vi "Client Single Connection.vi"() -> ()   [LabVIEW 2020]
doc: "This WebSockets API example VI acts as a client to make an outgoing websockets connection. Receives/sends string data to the connected server.\nWebSockets 2.0.1.40\nSam Sharp - MediaMongrels Ltd\nCopyright (c) 2019, MediaMongrels Ltd"
uses:
  <vilib>/MediaMongrels Ltd/WebSockets/WebSockets/WebSocket/WebSocket.lvclass/WebSocket.ctl
  <vilib>/MediaMongrels Ltd/WebSockets/WebSockets/WebSocket Client/WebSocket Client.lvclass
  C:/Program Files (x86)/National Instruments/LabVIEW 2020/vi.lib/MediaMongrels Ltd/WebSockets/WebSockets/WebSocket/WebSocket.lvclass
  <vilib>/MediaMongrels Ltd/WebSockets/WebSockets/WebSocket/WebSocket.lvclass
  <vilib>/addons/_JKI.lib/Serialization/JSON/JKI JSON Serialization.lvlib
panel:
  out "value":string
  in  "path":string[](array[string])
  in  "data":variant caption="Data"
  in  "command":string caption="Command"
  in  "Disconnect":bool
  in  "Connect":bool
  in  "WebSockets URL":string="ws://IP Address:Port"
  out "HTTP Headers":variant
  in  "Stop":bool
  out "Received Data":string
  in  "Send":bool
  # "WebSockets Client Example"
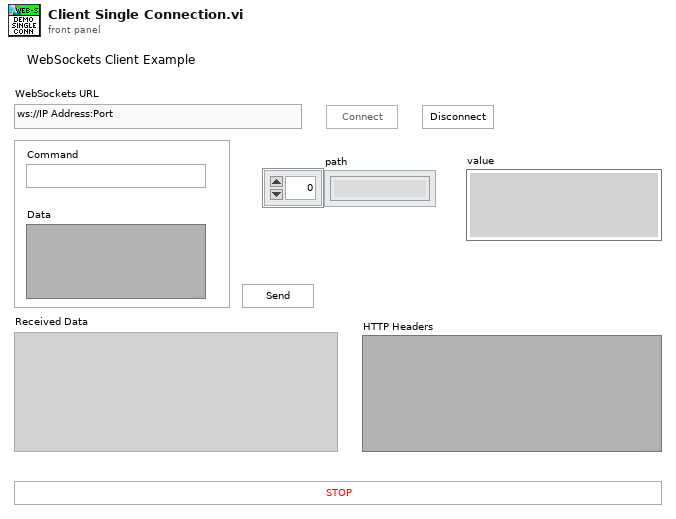
[diagram p1: front panel]
types:
  T1 = enum8{"Enabled", "Disabled", "Disabled and Grayed Out"}
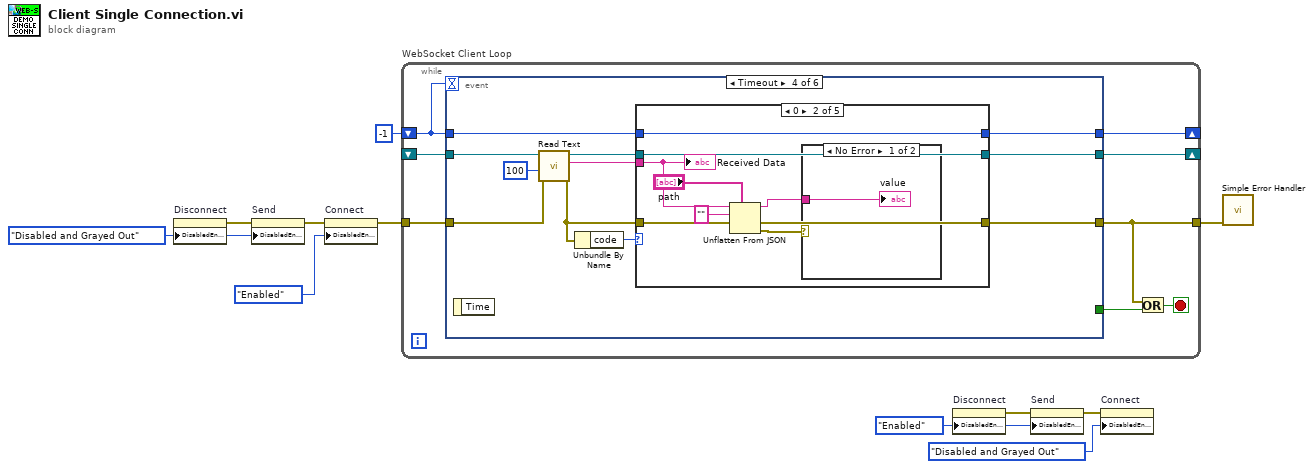
[diagram p0: block diagram]
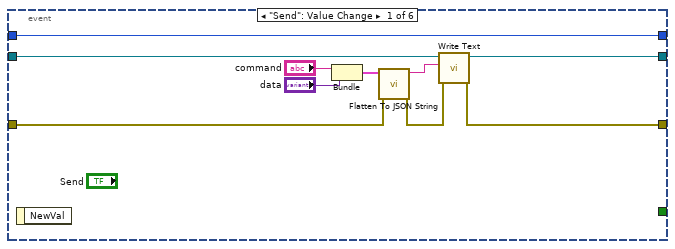
[diagram p2: hidden frame]
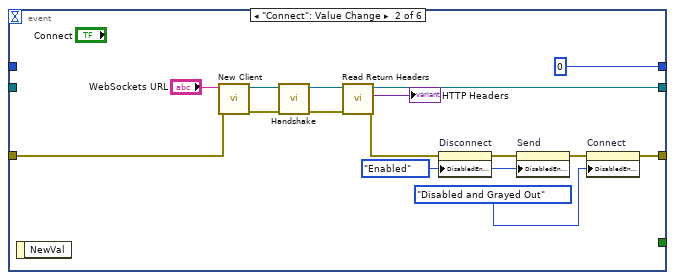
[diagram p3: hidden frame]
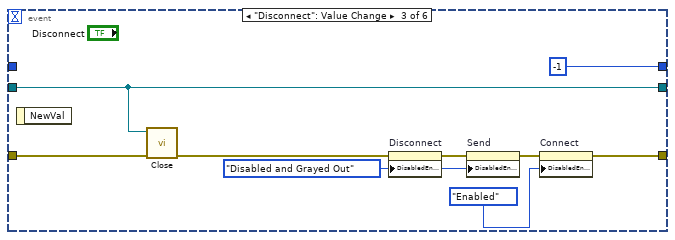
[diagram p4: hidden frame]
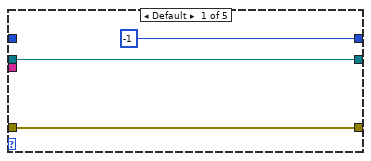
[diagram p5: hidden frame]
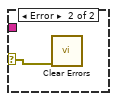
[diagram p6: hidden frame]
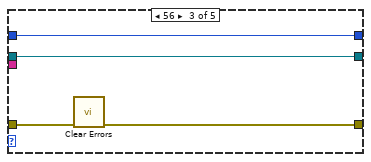
[diagram p7: hidden frame]
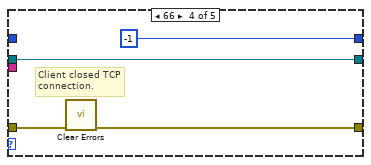
[diagram p8: hidden frame]
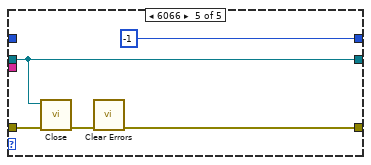
[diagram p9: hidden frame]
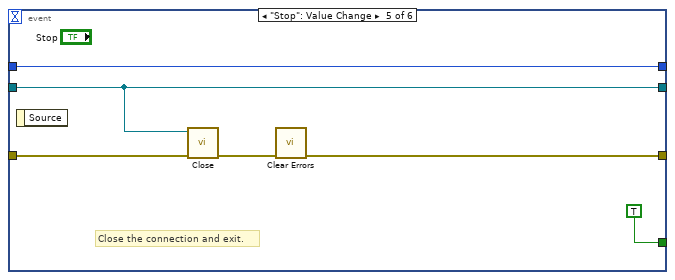
[diagram p10: hidden frame]
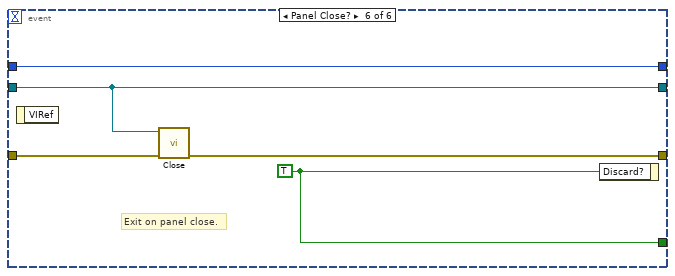
[diagram p11: hidden frame]
diagram:
  w4 = T1."Enabled" ("Disabled")
  w8 = T1."Disabled and Grayed Out" ("Disabled")
  n1 = property on="Disconnect" class="Bool"("DisabledEnum"=w8) -> (error out=w9:errorcluster)  [unwired: 2 in, 1 out]
  n2 = property on="Send" class="Bool"(error in=w9, "DisabledEnum"=w8) -> (error out=w3:errorcluster)  [unwired: 1 in, 1 out]
  n3 = property on="Connect" class="Bool"(error in=w3, "DisabledEnum"=T1."Enabled" ("Disabled")) -> (error out=w2:errorcluster)  [unwired: 1 in, 1 out]
  n4 = while "WebSocket Client Loop" {
    tunnel: [w16] -> w11
    tunnel: w2 -> [w19]
    shift-right: [w15] -> _
    shift-left: _ -> [w14]
    shift-right: [w13] -> _
    shift-left: -1 -> [w12]
    stop <- w17 stop-if-true
    n5 = event shown="[3] Timeout" {
      selector: _ -> [_ _ _ _ _ _]
      dyn-events: _ -> [_ _ _ _ _ _]
      timeout: w12 -> [_ _ _ _ _ _]
      tunnel: [_ _ _ _ TRUE w101] -> w18
      tunnel: [w29 w31 w45 w60 w91 w99] -> w16
      tunnel: w19 -> [w21 w43 w53 w64 w95 w100]
      tunnel: [w27 w38 w52 w57 w93 w98] -> w15
      tunnel: w14 -> [w28 _ w52 w63 w93 w98]
      tunnel: w12 -> [w26 _ _ w56 w92 w97]
      tunnel: [w26 0 -1 w55 w92 w97] -> w13
      event "Send": Value Change {
        n6 = event-data() -> ()  [unwired: 1 in, 1 out]
        n7 = Bundle("command"="command", "data"="data") -> (w24:cluster{"command":string, "data":variant})  [unwired: 1 in]
        n8 = call <vilib>:"Flatten To JSON String.vi"("error in (no error)"=w21, "Variant"=w24) -> ("error out"=w20:errorcluster, "JSON String"=w25:string)  [unwired: 8 in]
        n9 = call-dynamic "Write Text.vi"("error in (no error)"=w20, "String Data"=w25, "WebSocket in"=w28) -> ("error out"=w29:errorcluster, "WebSocket out"=w27:refnum<class "WebSocket Client.lvclass">)  [unwired: 7 in]
      }
      event "Connect": Value Change {
        w35 = T1."Enabled" ("Disabled")
        n10 = event-data() -> ()  [unwired: 1 in, 1 out]
        n11 = call <vilib>:"New Client.vi"("error in (no error)"=w43, "WebSocket URL"="WebSockets URL") -> ("error out"=w44:errorcluster, "WebSocket Client out"=w41:refnum<class "WebSocket Client.lvclass">)  [unwired: 8 in]
        n12 = call-dynamic "Handshake.vi"("error in (no error)"=w44, "WebSocket Client in"=w41) -> ("error out"=w40:errorcluster, "WebSocket Client out"=w39:refnum<class "WebSocket Client.lvclass">)  [unwired: 8 in]
        n13 = call <vilib>:"Read Return Headers.vi"("error in (no error)"=w40, "WebSocket in"=w39) -> ("error out"=w33:errorcluster, "Return Headers"=→"HTTP Headers":variant, "WebSocket out"=w38:refnum<class "WebSocket Client.lvclass">)  [unwired: 7 in]
        n14 = property on="Disconnect" class="Bool"(error in=w33, "DisabledEnum"=w35) -> (error out=w34:errorcluster)  [unwired: 1 in, 1 out]
        n15 = property on="Send" class="Bool"(error in=w34, "DisabledEnum"=w35) -> (error out=w32:errorcluster)  [unwired: 1 in, 1 out]
        n16 = property on="Connect" class="Bool"(error in=w32, "DisabledEnum"=T1."Disabled and Grayed Out" ("Disabled")) -> (error out=w31:errorcluster)  [unwired: 1 in, 1 out]
      }
      event "Disconnect": Value Change {
        w48 = T1."Disabled and Grayed Out" ("Disabled")
        n17 = event-data() -> ()  [unwired: 1 in, 1 out]
        n18 = call-dynamic "Close.vi"("error in (no error)"=w53, "WebSocket in"=w52) -> ("error out"=w46:errorcluster)  [unwired: 9 in]
        n19 = property on="Disconnect" class="Bool"(error in=w46, "DisabledEnum"=w48) -> (error out=w47:errorcluster)  [unwired: 1 in, 1 out]
        n20 = property on="Send" class="Bool"(error in=w47, "DisabledEnum"=w48) -> (error out=w49:errorcluster)  [unwired: 1 in, 1 out]
        n21 = property on="Connect" class="Bool"(error in=w49, "DisabledEnum"=T1."Enabled" ("Disabled")) -> (error out=w45:errorcluster)  [unwired: 1 in, 1 out]
      }
      event Timeout {
        n22 = event-data() -> ()  [unwired: 1 in, 1 out]
        n23 = call-dynamic "Read Text.vi"("error in (no error)"=w64, "timeout ms (5000)"=100, "WebSocket in"=w63) -> ("error out"=w59:errorcluster, "Data"=w54:string, "WebSocket out"=w58:refnum<class "WebSocket Client.lvclass">)  [unwired: 6 in]
        n24 = Unbundle By Name(w59) -> ("code"=w61:i32)
        n25 = case shown="0" w61 {
          tunnel: w54 -> [_ w68 _ _ _]
          tunnel: [w67 w75 w80 w82 w86] -> w60
          tunnel: w59 -> [w67 w75 w81 w85 w90]
          tunnel: w58 -> [w66 w74 w79 w84 w88]
          tunnel: [w66 w74 w79 w84 w88] -> w57
          tunnel: w56 -> [_ w73 w78 _ _]
          tunnel: [-1 w73 w78 -1 -1] -> w55
          frame Default {
          }
          frame 0 {
            n26 = Unflatten From JSON(path="path", JSON string=w68, type and defaults="") -> (value=w69:string, error out=w70:errorcluster)  [unwired: 4 in]
            n27 = case shown="No Error" w70 {
              selector: w70 -> [_ w77]
              tunnel: w69 -> [w76 _]
              frame No Error {
                "value" <- w76
              }
              frame Error {
                n28 = call <vilib>:"Clear Errors.vi"("error in (no error)"=w77) -> ()  [unwired: 5 in, 2 out]
              }
            }
            "Received Data" <- w68
          }
          frame 56 {
            n29 = call <vilib>:"Clear Errors.vi"("error in (no error)"=w81) -> ("error out"=w80:errorcluster)  [unwired: 5 in, 1 out]
          }
          frame 66 {
            # "Client closed TCP connection."
            n30 = call <vilib>:"Clear Errors.vi"("error in (no error)"=w85) -> ("error out"=w82:errorcluster)  [unwired: 5 in, 1 out]
          }
          frame 6066 {
            n31 = call-dynamic "Close.vi"("error in (no error)"=w90, "WebSocket in"=w88) -> ("error out"=w89:errorcluster)  [unwired: 9 in]
            n32 = call <vilib>:"Clear Errors.vi"("error in (no error)"=w89) -> ("error out"=w86:errorcluster)  [unwired: 5 in, 1 out]
          }
        }
      }
      event "Stop": Value Change {
        # "Close the connection and exit."
        n33 = event-data() -> ()  [unwired: 1 in, 1 out]
        n34 = call-dynamic "Close.vi"("error in (no error)"=w95, "WebSocket in"=w93) -> ("error out"=w94:errorcluster)  [unwired: 9 in]
        n35 = call <vilib>:"Clear Errors.vi"("error in (no error)"=w94) -> ("error out"=w91:errorcluster)  [unwired: 5 in, 1 out]
      }
      event Panel Close? {
        w101 = TRUE ("Discard?")
        # "Exit on panel close."
        n36 = event-data() -> ()  [unwired: 1 in, 1 out]
        n37 = call-dynamic "Close.vi"("error in (no error)"=w100, "WebSocket in"=w98) -> ("error out"=w99:errorcluster)  [unwired: 9 in]
        n38 = event-data("Discard?"=w101) -> ()  [unwired: 1 in, 1 out]
      }
    }
    n39 = Or(x=w16, y=w18) -> (x .or. y?=w17:bool)
  }
  n40 = property on="Disconnect" class="Bool"("DisabledEnum"=w4) -> (error out=w5:errorcluster)  [unwired: 2 in, 1 out]
  n41 = property on="Send" class="Bool"(error in=w5, "DisabledEnum"=w4) -> (error out=w6:errorcluster)  [unwired: 1 in, 1 out]
  n42 = property on="Connect" class="Bool"(error in=w6, "DisabledEnum"=T1."Disabled and Grayed Out" ("Disabled")) -> ()  [unwired: 1 in, 2 out]
  n43 = call <vilib>:"Simple Error Handler.vi"("error in (no error)"=w11) -> ()  [unwired: 4 in, 5 out]
